vi "Run Top Level.vi"(6 "Run/Open (T = Run)":bool=TRUE, 8 "error in":errorcluster, 10 "Project Reference":refnum<vi>) -> (0 "error out":errorcluster)   [LabVIEW 2020]
doc: "Run the top level VI in the project."
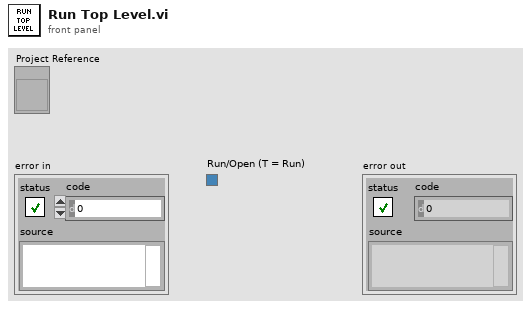
[diagram p1: front panel]
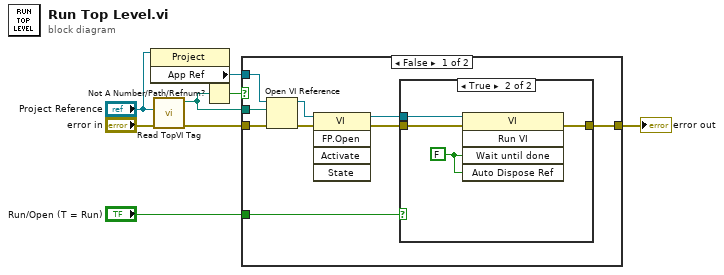
[diagram p0: block diagram]
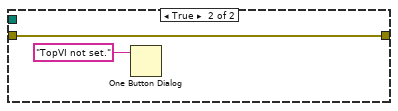
[diagram p3: hidden frame]
diagram:
  n1 = property class="Project"(reference="Project Reference") -> ("App Ref"=w2:refnum<vi>)  [unwired: 1 in, 2 out]
  n2 = call "Read TopVI Tag.vi"("error in"="error in", "Project Reference"="Project Reference") -> ("error out"=w6:errorcluster, "TopVI Path"=w5:path)  [unwired: 7 in, 1 out]
  n3 = Not A Number/Path/Refnum?(number/path/refnum=w5) -> (NaN/Path/Refnum?=w4:bool)
  n4 = case shown="False" w4 {
    tunnel: [w17 w24] -> w7
    tunnel: w6 -> [w16 w24]
    tunnel: w5 -> [w13 _]
    tunnel: w2 -> [w12 _]
    tunnel: "Run/Open (T = Run)" -> [w9 _]
    frame False {
      n5 = Open VI Reference(application reference (local)=w12, vi path=w13, error in (no error)=w16) -> (vi reference=w11:refnum<vi>, error out=w15:errorcluster)  [unwired: 3 in]
      n6 = invoke class="VI" method="FP.Open"(reference=w11, error in=w15) -> (reference out=w10:refnum<vi>, error out=w14:errorcluster)  [unwired: 3 in, 3 out]
      n7 = case shown="True" w9 {
        tunnel: [w18 w22] -> w17
        tunnel: w14 -> [w18 w21]
        tunnel: w10 -> [_ w19]
        frame False {
        }
        frame True {
          w20 = FALSE ("Auto Dispose Reference")
          n8 = invoke class="VI" method="Run VI"(reference=w19, error in=w21, "Wait until done"=w20, "Auto Dispose Ref"=w20) -> (error out=w22:errorcluster)  [unwired: 1 in, 4 out]
        }
      }
    }
    frame True {
      n9 = One Button Dialog(message="TopVI not set." ("t")) -> ()  [unwired: 1 in, 1 out]
    }
  }
  "error out" <- w7
